vi "HorseMantain.vi"(8 "Negative":bool, 9 "Positive":bool, 10 "HorseToggle":bool) -> (3 "Power":dbl)   [LabVIEW 2018]
uses:
  <vilib>/Rock Robotics/WPI/ThirdParty/Phoenix-LabVIEW/Motor Controller/Get/CTRE_Phoenix_MotorController_GetSelectedSensorData.vi
  <vilib>/addons/control/pid/pid.llb/PID (DBL).vi
  <vilib>/addons/control/pid/NI_PID_pid.lvlib
panel:
  out "Position (Raw Sensor Units)":i32
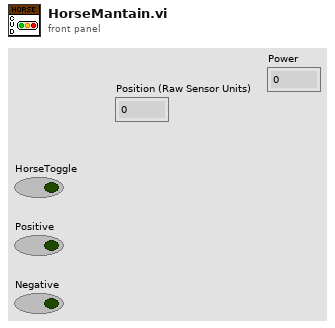
[diagram p1: front panel]
types:
  T1 = typedef "WPI_MotorControlDeviceRef.ctl" = cluster{"DeviceStatus":errorcluster, "Type":T2, "PWM":cluster{"PWM Channel":T3, "DeadBand":T4}, "CAN":cluster{"Device Number":u8, "SetOutput VI Ref":variant, "GetOutput VI Ref":variant, "Enable VI Ref":variant, "Disable VI Ref":variant, "Data":variant}, "Invert":bool, "DIO PWM":cluster{"PWM \"Enable\" Channel":T3, "DIOChannel":T5, "PWM Rate":dbl}}
  T2 = typedef "WPI_MotorControlType.ctl" = enum16{"PWM", "CAN", "DIO PWM"}
  T3 = typedef "FPGA_DIOPWMChannel.ctl" = enum8{"PWM 0", "PWM 1", "PWM 2", "PWM 3", "PWM 4", "PWM 5", "PWM 6", "PWM 7", "PWM 8", "PWM 9", "PWM MXP 0", "PWM MXP 1", "PWM MXP 2", "PWM MXP 3", "PWM MXP 4", "PWM MXP 5", "PWM MXP 6", "PWM MXP 7", "PWM MXP 8", "PWM MXP 9", "Invalid"}
  T4 = typedef "WPI_PWMDeadband.ctl" = cluster{"Name":string, "maxPositivePwm":i32, "minPositivePwm":i32, "centerPwm":i32, "maxNegativePwm":i32, "minNegativePwm":i32, "angularRange":u16}
  T5 = typedef "FPGA_DIOChannel.ctl" = enum8{"DIO 0", "DIO 1", "DIO 2", "DIO 3", "DIO 4", "DIO 5", "DIO 6", "DIO 7", "DIO 8", "DIO 9", "DIO MXP 0", "DIO MXP 1", "DIO MXP 2", "DIO MXP 3", "DIO MXP 4", "DIO MXP 5", "DIO MXP 6", "DIO MXP 7", "DIO MXP 8", "DIO MXP 9", "DIO MXP 10", "DIO MXP 11", "DIO MXP 12", "DIO MXP 13", "DIO MXP 14", "DIO MXP 15", "SPI Port CS1", "SPI Port CS2", "SPI Port CS3", "SPI Port MISO", "SPI Port MOSI", "Invalid"}
  T6 = cluster{"proportional gain (Kc)":dbl, "integral time (Ti, min)":dbl, "derivative time (Td, min)":dbl}
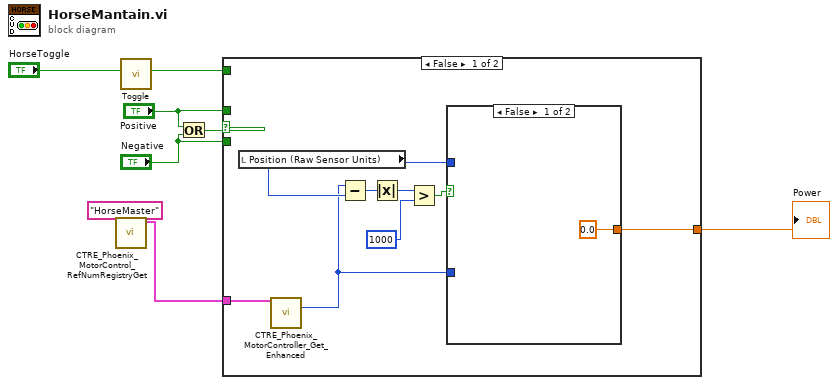
[diagram p0: block diagram]
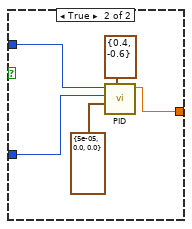
[diagram p2: hidden frame]
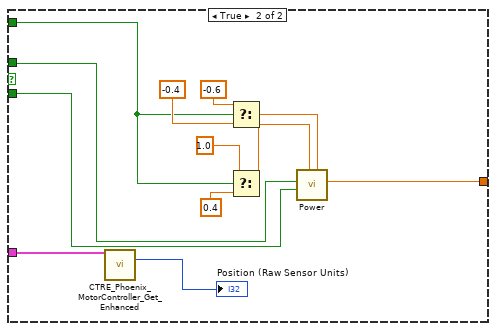
[diagram p3: hidden frame]
diagram:
  (unwired) "HorseMaster" ("refnum name")
  n1 = call <vilib>:"CTRE_Phoenix_MotorControl_RefNumRegistryGet.vi"() -> ("PhoenixMotorControlDevRef"=w4:T1)  [unwired: 10 in, 1 out]
  n2 = call "Toggle.vi"("Input"="HorseToggle") -> ("Output"=w6:bool)  [unwired: 10 in]
  n3 = Or(x="Positive", y="Negative") -> (x .or. y?=w1:bool)
  n4 = case shown="False" w1 {
    tunnel: "Positive" -> [_ w27]
    tunnel: "Negative" -> [_ w26]
    tunnel: [w14 w25] -> w5
    tunnel: w4 -> [w15 w24]
    tunnel: w6 -> [_ w22]
    frame False {
      n5 = local read "Position (Raw Sensor Units)"() -> (w13:i32)
      n6 = call-poly <vilib>:"CTRE_Phoenix_MotorController_Get_Enhanced.vi"("PhoenixMotorControlDevRef"=w15) -> ("Position (Raw Sensor Units)"=w12:i32)  [unwired: 11 in, 3 out]
      n7 = Subtract(x=w12, y=w13) -> (x-y=w11:i32)
      n8 = Absolute Value(x=w11) -> (abs(x)=w10:i32)
      n9 = Greater?(x=w10, y=1000) -> (0:w8:bool)
      n10 = case shown="False" w8 {
        tunnel: w12 -> [_ w19]
        tunnel: [0.0 ("output") w18] -> w14
        tunnel: w13 -> [_ w17]
        frame False {
        }
        frame True {
          n11 = call-poly <vilib>:"PID.vi"("output range"=cluster{"output high":dbl, "output low":dbl} {"output high"=0.4, "output low"=-0.6}, "PID gains"=T6 {"proportional gain (Kc)"=5e-05, "integral time (Ti, min)"=0.0, "derivative time (Td, min)"=0.0}, "process variable"=w19, "setpoint"=w17) -> ("output"=w18:dbl)  [unwired: 6 in, 1 out]
        }
      }
    }
    frame True {
      n12 = call-poly <vilib>:"CTRE_Phoenix_MotorController_Get_Enhanced.vi"("PhoenixMotorControlDevRef"=w24) -> ("Position (Raw Sensor Units)"=→"Position (Raw Sensor Units)":i32)  [unwired: 11 in, 3 out]
      n13 = Select(t=-0.6 ("f"), s=w22, f=-0.4) -> (s? t:f=w31:dbl)
      n14 = Select(t=1.0 ("f"), s=w22, f=0.4) -> (s? t:f=w30:dbl)
      n15 = call "Power.vi"("Negative Power"=w31, "Positive Power"=w30, "Negative"=w26, "Positive"=w27) -> ("Output"=w25:dbl)  [unwired: 7 in]
    }
  }
  "Power" <- w5
